vi "Tecan Start.vi"(0 "VISA resource name":refnum<visa-resource-name>="COM3", 1 "Pump Address":T2, 2 "Abs":bool, 5 "Direction":T3, 7 "Rate(uL/min)":dbl, 9 "Volume(uL)":dbl, 11 "error IO":errorcluster, 12 "Syringe Capacity":dbl) -> (4 "VISA resource name out":refnum<visa-resource-name>, 6 "Current Position(mL)":u32, 8 "Error Code":string, 10 "Move Successful":bool, 14 "Response":string, 15 "error out":errorcluster)   [LabVIEW 2018]
uses:
  Pump Direction.ctl
  Pump Address.ctl
  Velocity Units.ctl
  Hardware Globals.vi
panel:
  in  "Units":T1
  out "Current Position(steps)":u32 caption="Current Position(half steps)"
  # "range:  0-15000 ul/min"
  # "range:  0-2000"
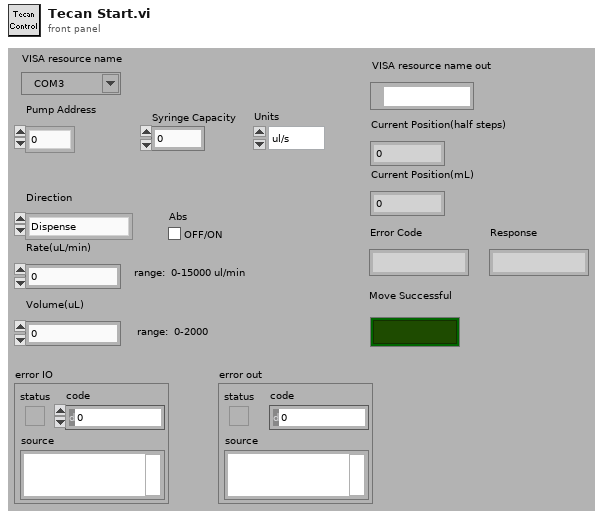
[diagram p1: front panel]
types:
  T1 = typedef "Velocity Units.ctl" = enum16{"ul/s", "ul/min"}
  T2 = typedef "Pump Address.ctl" = enum16{"0", "1", "2", "3", "4", "5", "6", "7"}
  T3 = typedef "Pump Direction.ctl" = enum16{"Dispense", "Withdraw", "Stop"}
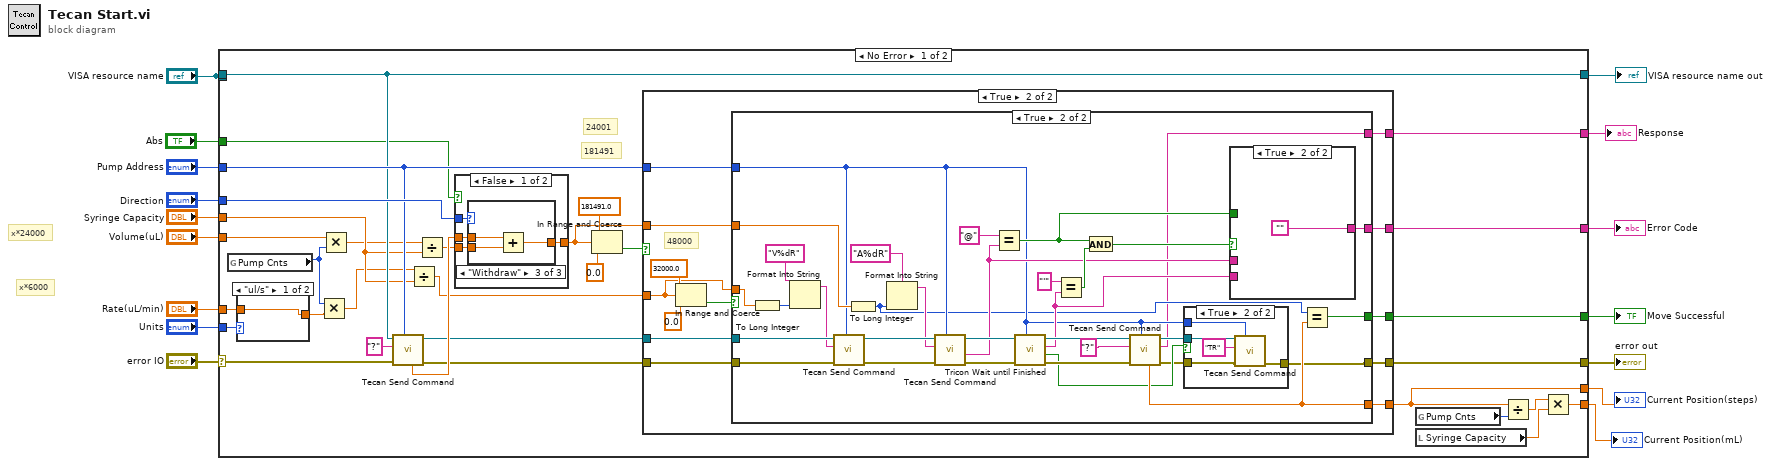
[diagram p0: block diagram]
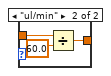
[diagram p2: hidden frame]
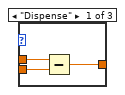
[diagram p3: hidden frame]
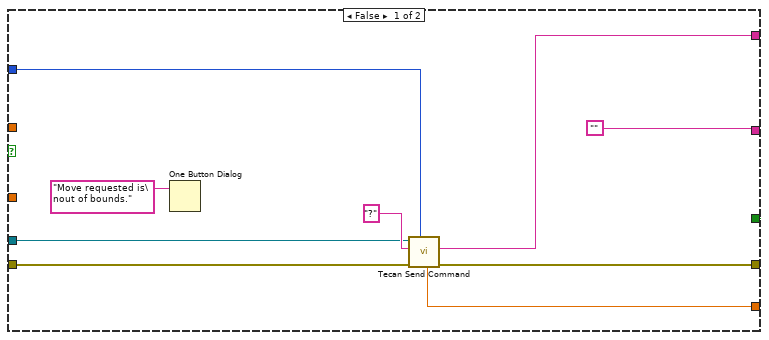
[diagram p6: hidden frame]
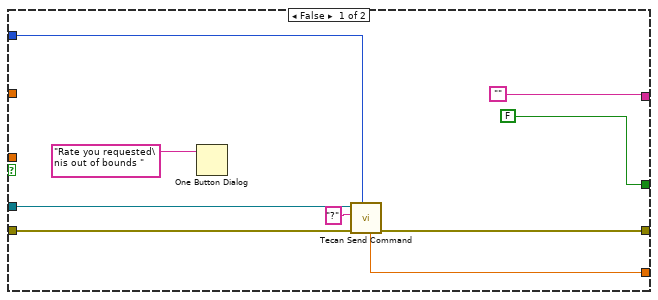
[diagram p7: hidden frame]
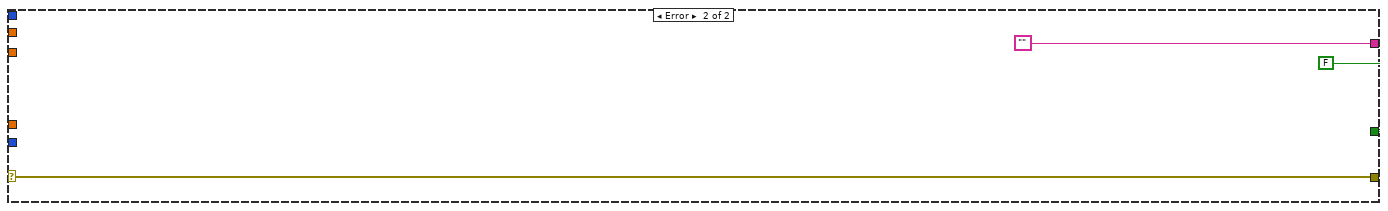
[diagram p11: hidden frame]
diagram:
  # "x*24000"
  # "x*6000"
  n1 = case shown="No Error" "error IO" {
    selector: "error IO" -> [w47 w145]
    tunnel: [w48 w145] -> w16
    tunnel: "VISA resource name" -> [_ _]
    tunnel: "Volume(uL)" -> [w22 _]
    tunnel: "Rate(uL/min)" -> [w23 _]
    tunnel: "Direction" -> [w45 _]
    tunnel: "Pump Address" -> [w35 _]
    tunnel: "VISA resource name" -> [w34 _]
    tunnel: [w37 FALSE] -> w9
    tunnel: [w30 _] -> w4
    tunnel: [w36 ""] -> w8
    tunnel: [w34 _] -> w7
    tunnel: "Syringe Capacity" -> [w32 _]
    tunnel: [w27 _] -> w5
    tunnel: [w26 _] -> w3
    tunnel: "Abs" -> [w25 _]
    tunnel: "Units" -> [w24 _]
    frame No Error {
      # "181491"
      # "24001"
      n2 = global read "Hardware Globals.vi" "Pump Cnts"() -> (w18:i32)
      n3 = case shown="\"ul/s\"" w24 {
        tunnel: w23 -> [w49 w52]
        tunnel: [w49 w50] -> w21
        frame "ul/s" {
        }
        frame "ul/min" {
          n4 = Divide(x=w52, y=60.0) -> (x/y=w50:dbl)
        }
      }
      n5 = Multiply(x=w18, y=w21) -> (x*y=w20:dbl)
      n6 = Multiply(x=w22, y=w18) -> (x*y=w19:dbl)
      n7 = call "Tecan Send Command.vi"("Address"=w35, "error in (no error)"=w47, "Command"="?", "VISA resource name in"=w34) -> ("error out"=w40:errorcluster, "VISA resource name out"=w39:refnum<visa-resource-name>, "Value"=w44:dbl)  [unwired: 3 in, 2 out]
      n8 = Divide(x=w20, y=w32) -> (x/y=w31:dbl)
      n9 = Divide(x=w19, y=w32) -> (x/y=w33:dbl)
      n10 = case shown="False" w25 {
        tunnel: w45 -> [w56 _]
        tunnel: w44 -> [w55 _]
        tunnel: [w54 w64] -> w38
        tunnel: w33 -> [w53 w64]
        frame False {
          n11 = case shown="\"Withdraw\"" w56 {
            tunnel: w53 -> [w57 _ w61]
            tunnel: [w59 w60 w63] -> w54
            tunnel: w55 -> [w58 w60 w62]
            frame "Dispense" {
              n12 = Subtract(x=w58, y=w57) -> (x-y=w59:dbl)
            }
            frame "Stop" {
            }
            frame "Withdraw" {
              n13 = Add(x=w62, y=w61) -> (x+y=w63:dbl)
            }
          }
        }
        frame True {
        }
      }
      n14 = In Range and Coerce(upper limit=181491.0, x=w38, lower limit=0.0 ("upper limit")) -> (In Range?=w41:bool)  [unwired: 1 out]
      n15 = case shown="True" w41 {
        tunnel: [w70 w87] -> w48
        tunnel: w40 -> [w71 w86]
        tunnel: w35 -> [w66 w85]
        tunnel: w39 -> [w69 w84]
        tunnel: w31 -> [_ w76]
        tunnel: w38 -> [_ w80]
        tunnel: [FALSE w79] -> w37
        tunnel: [w68 w78] -> w27
        tunnel: ["" w77] -> w36
        tunnel: [w65 w75] -> w26
        frame False {
          n16 = One Button Dialog(message="Move requested is\nout of bounds.") -> ()  [unwired: 1 in, 1 out]
          n17 = call "Tecan Send Command.vi"("Address"=w66, "error in (no error)"=w71, "Command"="?", "VISA resource name in"=w69) -> ("error out"=w70:errorcluster, "Raw Response"=w65:string, "Value"=w68:dbl)  [unwired: 3 in, 2 out]
        }
        frame True {
          # "48000"
          n18 = In Range and Coerce(upper limit=32000.0, x=w76, lower limit=0.0) -> (In Range?=w81:bool)  [unwired: 1 out]
          n19 = case shown="True" w81 {
            tunnel: [w92 w99] -> w87
            tunnel: w86 -> [w93 w129]
            tunnel: w85 -> [w88 w101]
            tunnel: w84 -> [w91 w128]
            tunnel: w76 -> [_ w126]
            tunnel: w80 -> [_ w122]
            tunnel: [FALSE w113] -> w79
            tunnel: [w90 w112] -> w78
            tunnel: ["" w107] -> w77
            tunnel: [_ w97] -> w75
            frame False {
              n20 = One Button Dialog(message="Rate you requested\nis out of bounds ") -> ()  [unwired: 1 in, 1 out]
              n21 = call "Tecan Send Command.vi"("Address"=w88, "error in (no error)"=w93, "Command"="?", "VISA resource name in"=w91) -> ("error out"=w92:errorcluster, "Value"=w90:dbl)  [unwired: 3 in, 3 out]
            }
            frame True {
              # "`"
              n22 = To Long Integer(number=w126) -> (32bit integer=w125:i32)
              n23 = Format Into String(format string="V%dR", w125) -> (resulting string=w123:string)  [unwired: 2 in, 1 out]
              n24 = call "Tecan Send Command.vi"("Address"=w101, "error in (no error)"=w129, "Command"=w123, "VISA resource name in"=w128) -> ("error out"=w124:errorcluster, "VISA resource name out"=w120:refnum<visa-resource-name>)  [unwired: 3 in, 3 out]
              n25 = To Long Integer(number=w122) -> (32bit integer=w100:i32)
              n26 = Format Into String(format string="A%dR", w100) -> (resulting string=w119:string)  [unwired: 2 in, 1 out]
              n27 = call "Tecan Send Command.vi"("Address"=w101, "error in (no error)"=w124, "Command"=w119, "VISA resource name in"=w120) -> ("error out"=w117:errorcluster, "Status Code"=w104:string, "VISA resource name out"=w118:refnum<visa-resource-name>)  [unwired: 3 in, 2 out]
              n28 = Equal?(x="@", y=w104) -> (x = y?=w106:bool)
              n29 = call "Tricon Wait until Finished.vi"("Pump Address"=w101, "error out"=w117, "VISA resource name in"=w118) -> ("error out"=w114:errorcluster, "Cancelled"=w103:bool, "Error Code"=w105:string, "VISA resource name out"=w115:refnum<visa-resource-name>)  [unwired: 5 in]
              n30 = Equal?(x="'", y=w105) -> (x = y?=w109:bool)
              n31 = And(x=w106, y=w109) -> (x .and. y?=w108:bool)
              n32 = call "Tecan Send Command.vi"("Address"=w101, "error in (no error)"=w114, "Command"="?", "VISA resource name in"=w115) -> ("error out"=w102:errorcluster, "Raw Response"=w97:string, "VISA resource name out"=w98:refnum<visa-resource-name>, "Value"=w112:dbl)  [unwired: 3 in, 1 out]
              n33 = case shown="True" w103 {
                tunnel: w102 -> [w130 w135]
                tunnel: w101 -> [_ w133]
                tunnel: [w130 w132] -> w99
                tunnel: w98 -> [_ w131]
                frame False {
                }
                frame True {
                  n34 = call "Tecan Send Command.vi"("Address"=w133, "error in (no error)"=w135, "Command"="TR", "VISA resource name in"=w131) -> ("error out"=w132:errorcluster)  [unwired: 3 in, 4 out]
                }
              }
              n35 = case shown="True" w108 {
                tunnel: [w138 ""] -> w107
                tunnel: w106 -> [w139 _]
                tunnel: w105 -> [w137 _]
                tunnel: w104 -> [w136 _]
                frame False {
                  n36 = case shown="False" w139 {
                    tunnel: [w140 w141] -> w138
                    tunnel: w137 -> [_ w141]
                    tunnel: w136 -> [w140 _]
                    frame False {
                    }
                    frame True {
                    }
                  }
                }
                frame True {
                }
              }
              n37 = Equal?(x=w100, y=w112) -> (x = y?=w113:bool)
            }
          }
        }
      }
      n38 = global read "Hardware Globals.vi" "Pump Cnts"() -> (w17:i32)
      n39 = local read "Syringe Capacity"() -> (w28:dbl)
      n40 = Divide(x=w27, y=w17) -> (x/y=w29:dbl)
      n41 = Multiply(x=w29, y=w28) -> (x*y=w30:dbl)
    }
    frame Error {
    }
  }
  "error out" <- w16
  "VISA resource name out" <- w7
  "Move Successful" <- w9
  "Current Position(steps)" <- w5
  "Error Code" <- w8
  "Current Position(mL)" <- w4
  "Response" <- w3
